vi "niRFUtil RFHS Benchmark Enter.vi"(5 "ID Changed":bool, 7 "ID":string, 9 "error in (no error)":errorcluster, 11 "Benchmark Task (Parent)":T1) -> (1 "error out":errorcluster, 3 "Benchmark Task (Self)":T1)   [LabVIEW 2015, in "niRFUtil.lvlib"]
uses:
  niRFUtil.lvlib
  niRFUtil RFHS Benchmark Task.ctl
  niRFUtil RFHS Util Phases.ctl
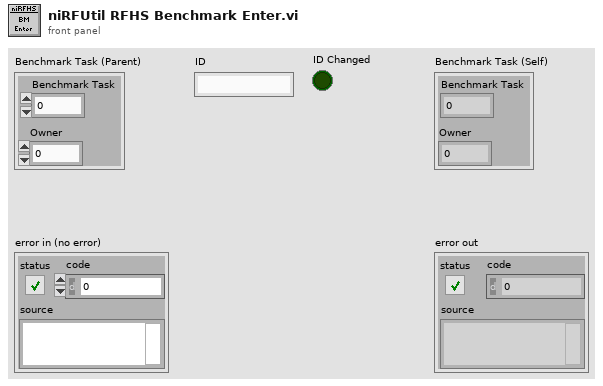
[diagram p1: front panel]
types:
  T1 = typedef "niRFUtil.lvlib/niRFUtil RFHS Benchmark Task.ctl" = cluster{"Benchmark Task":u64, "Owner":u32}
  T2 = typedef "niRFUtil.lvlib/niRFUtil RFHS Util Phases.ctl" = enum32{"Reserved", "CreateBenchmarkTask", "CRC", "UE UL Segment Transport Block", "UE UL Read Buffer", "UE UL TC", "UE UL RM", "UE UL CI", "Scramble", "Group Bits", "Benchmark Task Start", "Benchmark Task Stop", "Descramble", "Deinterleave", "eNB UL HARQ", "eNB UL Read Buffer", "eNB UL AFEM", "eNB UL Turbo Decoder", "Get Benchmark Task Data", "G31", "UL Gen Freq2Time", "Gen Power Spectrum", "UL Ana Time2Freq", "Benchmark Task Enter", "Benchmark Task Leave"}
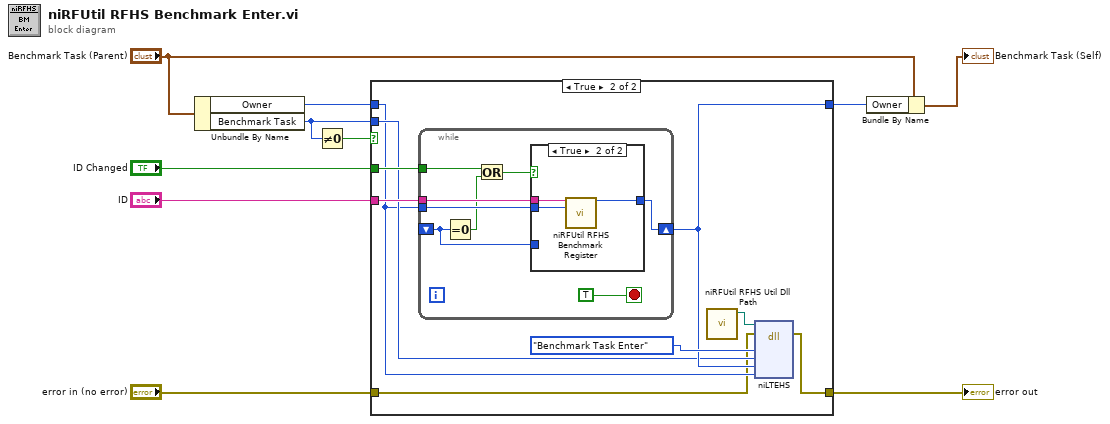
[diagram p0: block diagram]
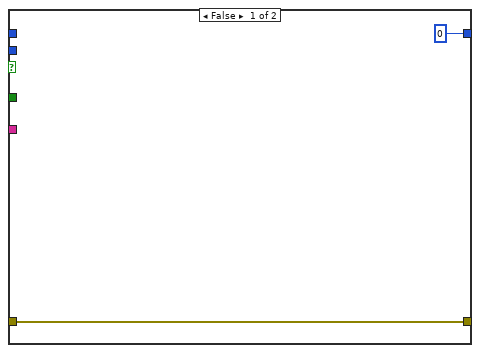
[diagram p2: hidden frame]
diagram:
  n1 = Unbundle By Name("Benchmark Task (Parent)") -> ("Owner"=w3:u32, "Benchmark Task"=w4:u64)
  n2 = Not Equal To 0?(x=w4) -> (x != 0?=w10:bool)
  n3 = case shown="True" w10 {
    tunnel: [u32 0 ("ID") w17] -> w7
    tunnel: "ID Changed" -> [_ w19]
    tunnel: "ID" -> [_ w18]
    tunnel: w4 -> [_ w16]
    tunnel: w3 -> [_ w15]
    tunnel: "error in (no error)" -> [w12 w14]
    tunnel: [w12 w13] -> w1
    frame False {
    }
    frame True {
      n4 = while {
        shift-right: [w28] -> w17
        shift-left: _ -> [w29]
        tunnel: w19 -> [w24]
        tunnel: w18 -> [w26]
        tunnel: w15 -> [w25]
        stop <- TRUE stop-if-true
        n5 = Equal To 0?(x=w29) -> (x = 0?=w23:bool)
        n6 = Or(x=w24, y=w23) -> (x .or. y?=w27:bool)
        n7 = case shown="True" w27 {
          tunnel: w29 -> [w30 _]
          tunnel: [w30 w33] -> w28
          tunnel: w26 -> [_ w32]
          tunnel: w25 -> [_ w31]
          frame False {
          }
          frame True {
            n8 = call "niRFUtil RFHS Benchmark Register.vi"("Special ID"=w32, "Owner"=w31) -> ("ID"=w33:u32)  [unwired: 13 in]
          }
        }
      }
      n9 = call "niRFUtil RFHS Util Dll Path.vi"() -> ("Path"=w21:path)  [unwired: 7 in, 4 out]
      n10 = dll-call lib="?" fn="niLTEHS"(path in=w21, error in=w14, "what"=niRFUtil_RFHS_Util_Phases."Benchmark Task Enter" ("Enum"), "benchmarkTask"=w16, "benchId"=w17, "owner"=w15) -> (error out=w13:errorcluster)  [unwired: 6 in, 1 out]
    }
  }
  "error out" <- w1
  n11 = Bundle By Name(cluster="Benchmark Task (Parent)", "Owner"=w7) -> (→"Benchmark Task (Self)":T1)
